vi "Custom Device Express CORE.vi"(8 "error in":errorcluster, 11 "CDEW_MetaDataObj in":refnum<class "NIVS_CDEW_MetaDataObj.lvclass">) -> (0 "error out":errorcluster, 3 "CDEW_MetaDataObj out":refnum<class "NIVS_CDEW_MetaDataObj.lvclass">)   [LabVIEW 2026, in "NIVS_CDEW_MetaDataObj.lvclass"]
doc: "This VI is the Core VI for the Custom Device Wizard.\n\nWritten by:\nStephan Daunke\n\nDate:\n2014/01/27\n\nCompany:\nNational Instruments Germany GmbH"
uses:
  NIVS_CDEW_MetaDataObj.lvclass
  NIVS_CDEW_MetaDataObj.lvclass/NIVS_CDEW_MetaDataObj.ctl
  Support/XML Parser/XML Parser.lvlib
  <vilib>/AppBuilder/AB_API_Simple/NI_App_Builder_API.lvlib
  0d099170-2439-4ee0-9fc1-b5448e48b177.vi
  <vilib>/AppBuilder/AB_API_Simple/Build (path).vi
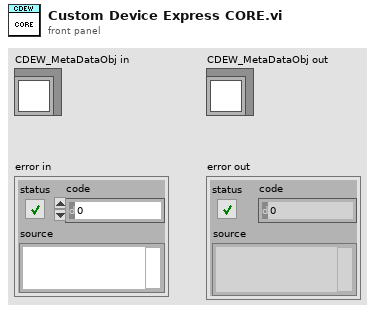
[diagram p1: front panel]
types:
  T1 = enum16{"Create CD Root Folder", "Copy Compiled Settings", "Generate Custom Device DLL from XML", "Calculate Page Properties", "Create Configuration Project", "Create Engine Project", "Create Custom Device Engine Project", "Create System Explorer Project", "Create Test Hooks Project", "Relink and Clean Up VIs", "Build PPLs", "Copy Custom Device DLL to Public Documents", "Open Projects"}
  T2 = enum16{"Create CD Root Folder", "Copy Compiled Settings", "Generate Custom Device DLL from XML", "Calculate Page Properties", "Create Configuration Project", "Create Engine Project", "Create Custom Device Engine Project", "Create System Explorer Project", "Create Test Hooks Project", "Relink and Clean Up VIs", "Build PPLs", "Copy Custom Device DLL to Public Documents", "Open Projects"}[]
  T3 = typedef "NIVS_CDEW_MetaDataObj.lvclass/Page Properties.ctl" = cluster{"Type":T4, "Name":string, "GUID":string, "PageDetail":string, "PageVIPath":path}
  T4 = typedef "NIVS_CDEW_MetaDataObj.lvclass/Page Types.ctl" = enum16{"None", "CustomDevice", "Channel", "Waveform", "Section", "DynamicChannel", "DynamicWaveform", "DynamicSection"}
  T5 = cluster{"Project":path, "Target":string, "BuildSpec":string}[]
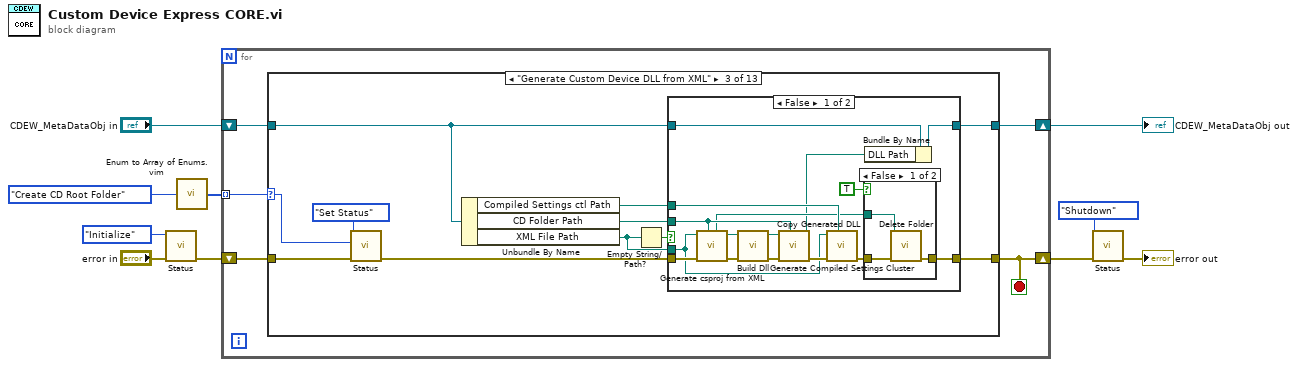
[diagram p0: block diagram]
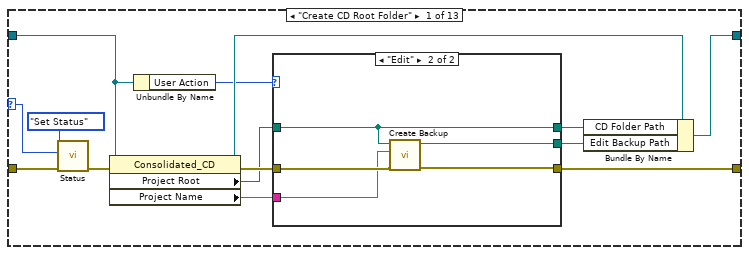
[diagram p2: hidden frame]
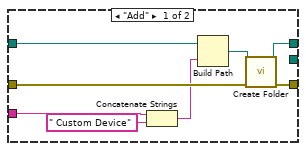
[diagram p3: hidden frame]
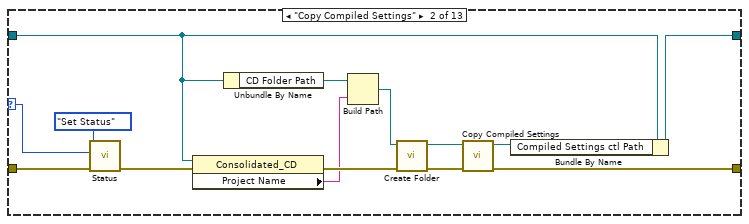
[diagram p4: hidden frame]
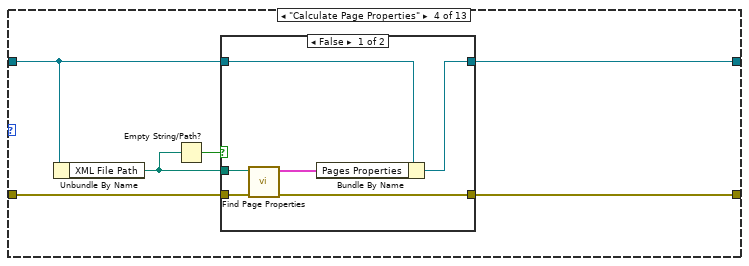
[diagram p7: hidden frame]
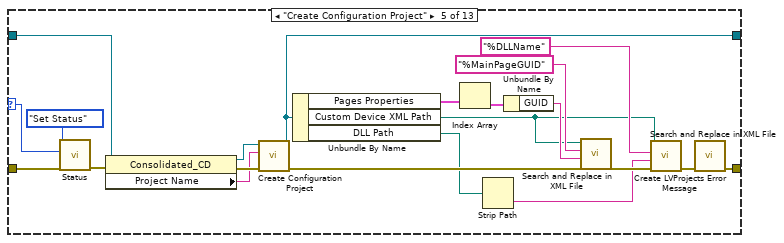
[diagram p9: hidden frame]
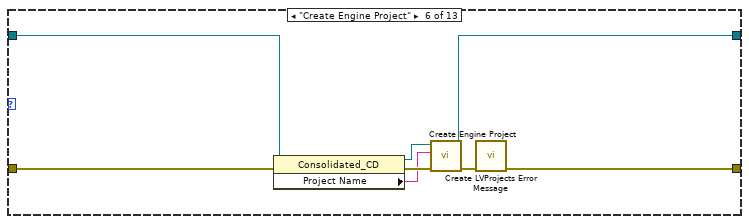
[diagram p10: hidden frame]
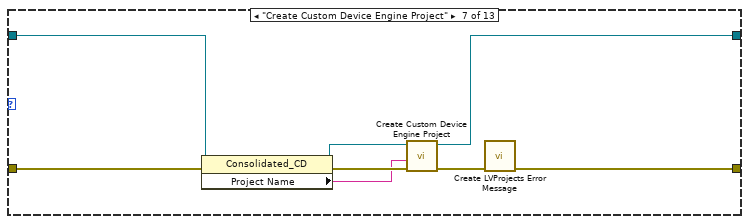
[diagram p11: hidden frame]
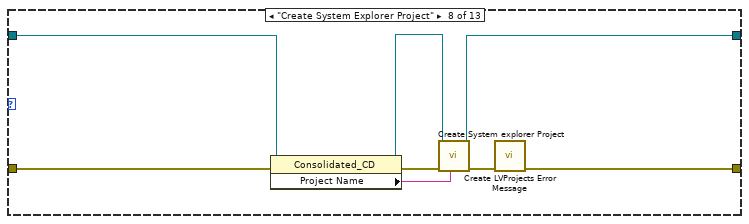
[diagram p12: hidden frame]
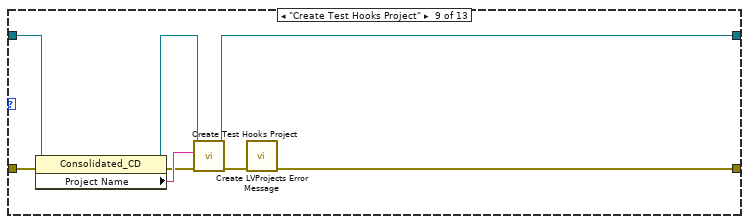
[diagram p13: hidden frame]
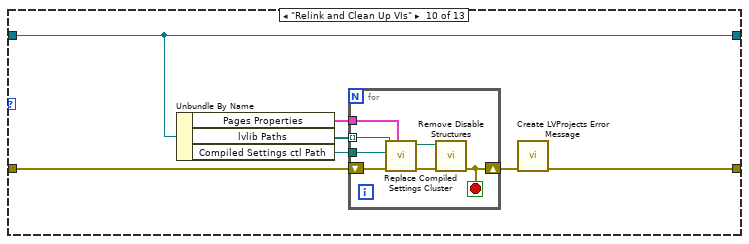
[diagram p14: hidden frame]
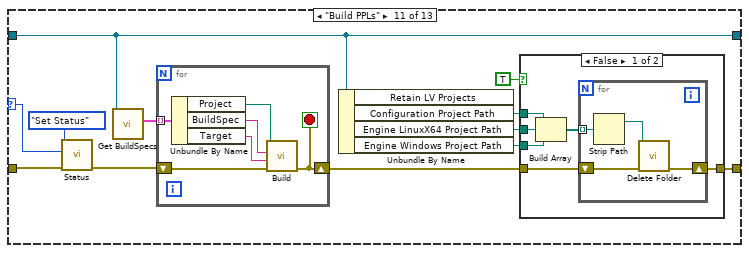
[diagram p15: hidden frame]
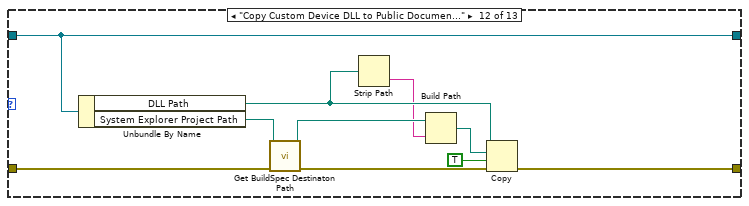
[diagram p17: hidden frame]
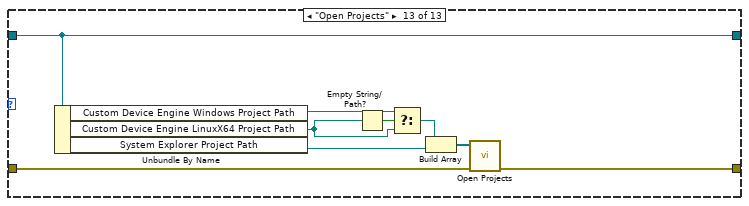
[diagram p18: hidden frame]
diagram:
  n1 = call "Status.vi"("error in"="error in", "Operation"=enum16{"Initialize", "Set Status", "Shutdown"}."Initialize") -> ("error out"=w9:errorcluster)  [unwired: 9 in]
  n2 = call "Enum to Array of Enums.vim"("enum"=T1."Create CD Root Folder") -> ("array of enums"=w1:T2)
  n3 = for {
    shift-right: [w14] -> w8
    shift-left: w9 -> [w15]
    shift-right: [w12] -> w5
    shift-left: "CDEW_MetaDataObj in" -> [w13]
    tunnel: w1 -> [w11] mode=indexing
    stop <- w14 stop-if-true
    n4 = case shown="\"Generate Custom Device DLL from XML\"" w11 {
      selector: w11 -> [w17 w44 w58 _ w105 _ _ _ _ _ w172 _ _]
      tunnel: w15 -> [w27 w53 w66 w95 w119 w131 w139 w147 w156 w163 w180 w207 w218]
      tunnel: [w29 w56 w67 w94 w120 w129 w137 w145 w155 w161 w182 w209 w217] -> w14
      tunnel: w13 -> [w22 w46 w61 w92 w112 w125 w135 w141 w151 w158 w177 w206 w216]
      tunnel: [w23 w51 w60 w93 w116 w127 w134 w143 w154 w158 w177 w206 w216] -> w12
      frame "Create CD Root Folder" {
        n5 = call "Status.vi"("error in"=w27, "State"=w17, "Operation"=enum16{"Initialize", "Set Status", "Shutdown"}."Set Status") -> ("error out"=w26:errorcluster)  [unwired: 8 in]
        n6 = property class="Consolidated_CD"(reference=w22, error in=w26) -> (reference out=w25:refnum<class "NIVS_CDEW_MetaDataObj.lvclass">, error out=w28:errorcluster, "Project Root"=w20:path, "Project Name"=w19:string)
        n7 = Unbundle By Name(w22) -> ("User Action"=w21:enum16{"Add", "Edit"})
        n8 = case shown="\"Edit\"" w21 {
          tunnel: [w37 w41] -> w29
          tunnel: [w35 w38] -> w24
          tunnel: w28 -> [w36 w42]
          tunnel: w20 -> [w33 w38]
          tunnel: w19 -> [w32 w40]
          tunnel: [_ w39] -> w18
          frame "Add" {
            n9 = Concatenate Strings(w32, " Custom Device" ("string")) -> (w30:string)
            n10 = Build Path(base path=w33, name or relative path=w30) -> (appended path=w34:path)
            n11 = call "Create Folder.vi"("error in"=w36, "Folder Path"=w34) -> ("error out"=w37:errorcluster, "Folder Path Out"=w35:path)  [unwired: 8 in]
          }
          frame "Edit" {
            n12 = call "Create Backup.vi"("error in"=w42, "Custom Device Name"=w40, "Custom Device Folder"=w38) -> ("error out"=w41:errorcluster, "Edit Backup Path"=w39:path)  [unwired: 7 in]
          }
        }
        n13 = Bundle By Name(cluster=w25, "CD Folder Path"=w24, "Edit Backup Path"=w18) -> (w23:refnum<class "NIVS_CDEW_MetaDataObj.lvclass">)
      }
      frame "Copy Compiled Settings" {
        n14 = call "Status.vi"("error in"=w53, "State"=w44, "Operation"=enum16{"Initialize", "Set Status", "Shutdown"}."Set Status") -> ("error out"=w52:errorcluster)  [unwired: 8 in]
        n15 = property class="Consolidated_CD"(reference=w46, error in=w52) -> (error out=w54:errorcluster, "Project Name"=w45:string)  [unwired: 1 out]
        n16 = Unbundle By Name(w46) -> ("CD Folder Path"=w49:path)
        n17 = Build Path(base path=w49, name or relative path=w45) -> (appended path=w48:path)
        n18 = call "Create Folder.vi"("error in"=w54, "Folder Path"=w48) -> ("error out"=w55:errorcluster, "Folder Path Out"=w47:path)  [unwired: 8 in]
        n19 = call "Copy Compiled Settings.vi"("error in"=w55, "Custom Device Folder"=w47) -> ("error out"=w56:errorcluster, "Compiled Settings ctl File Path"=w50:path)  [unwired: 8 in]
        n20 = Bundle By Name(cluster=w46, "Compiled Settings ctl Path"=w50) -> (w51:refnum<class "NIVS_CDEW_MetaDataObj.lvclass">)
      }
      frame "Generate Custom Device DLL from XML" {
        n21 = call "Status.vi"("error in"=w66, "State"=w58, "Operation"=enum16{"Initialize", "Set Status", "Shutdown"}."Set Status") -> ("error out"=w65:errorcluster)  [unwired: 8 in]
        n22 = Unbundle By Name(w61) -> ("Compiled Settings ctl Path"=w59:path, "CD Folder Path"=w62:path, "XML File Path"=w64:path)
        n23 = Empty String/Path?(string/path=w64) -> (empty?=w63:bool)
        n24 = case shown="False" w63 {
          tunnel: w65 -> [w83 w89]
          tunnel: [w78 w89] -> w67
          tunnel: w64 -> [w75 _]
          tunnel: w62 -> [w74 _]
          tunnel: w61 -> [w73 w88]
          tunnel: [w70 w88] -> w60
          tunnel: w59 -> [w72 _]
          frame False {
            n25 = call "Generate csproj from XML.vi"("CD Root Folder Path"=w74, "error in"=w83, "XML File Path"=w75) -> ("error out"=w81:errorcluster, "csproj Path"=w77:path, "CD Gen code folder"=w71:path)  [unwired: 6 in]
            n26 = call "Build Dll.vi"("error in"=w81, "csproj Path in"=w77) -> ("error out"=w82:errorcluster, "csproj Path out"=w76:path)  [unwired: 8 in]
            n27 = call "Copy Generated DLL.vi"("CD root folder Path"=w74, "error in"=w82, "csproj Path"=w76) -> ("error out"=w80:errorcluster, "CD DLL Path"=w69:path)  [unwired: 7 in]
            n28 = call "Generate Compiled Settings Cluster.vi"("Compiled Settings Path"=w72, "error in"=w80, "XML Path"=w75) -> ("error out"=w79:errorcluster)  [unwired: 8 in]
            n29 = case shown="False" TRUE {
              tunnel: w79 -> [w85 w87]
              tunnel: w71 -> [w84 _]
              tunnel: [w86 w87] -> w78
              frame False {
                n30 = call "Delete Folder.vi"("error in"=w85, "Folder Path"=w84) -> ("error out"=w86:errorcluster)  [unwired: 8 in, 1 out]
              }
              frame True {
              }
            }
            n31 = Bundle By Name(cluster=w73, "DLL Path"=w69) -> (w70:refnum<class "NIVS_CDEW_MetaDataObj.lvclass">)
          }
          frame True {
          }
        }
      }
      frame "Calculate Page Properties" {
        n32 = Unbundle By Name(w92) -> ("XML File Path"=w91:path)
        n33 = Empty String/Path?(string/path=w91) -> (empty?=w90:bool)
        n34 = case shown="False" w90 {
          tunnel: w95 -> [w101 w103]
          tunnel: [w100 w103] -> w94
          tunnel: w91 -> [w99 _]
          tunnel: [w97 w102] -> w93
          tunnel: w92 -> [w96 w102]
          frame False {
            n35 = call "Find Page Properties.vi"("error in"=w101, "XML File Path"=w99) -> ("error out"=w100:errorcluster, "Pages Properties"=w98:T3[])  [unwired: 8 in]
            n36 = Bundle By Name(cluster=w96, "Pages Properties"=w98) -> (w97:refnum<class "NIVS_CDEW_MetaDataObj.lvclass">)
          }
          frame True {
          }
        }
      }
      frame "Create Configuration Project" {
        n37 = call "Status.vi"("error in"=w119, "State"=w105, "Operation"=enum16{"Initialize", "Set Status", "Shutdown"}."Set Status") -> ("error out"=w118:errorcluster)  [unwired: 8 in]
        n38 = property class="Consolidated_CD"(reference=w112, error in=w118) -> (reference out=w113:refnum<class "NIVS_CDEW_MetaDataObj.lvclass">, error out=w124:errorcluster, "Project Name"=w117:string)
        n39 = call "Create Configuration Project.vi"("error in"=w124, "Custom Device Name"=w117, "CDEW_MetaDataObj in"=w113) -> ("error out"=w123:errorcluster, "CDEW_MetaDataObj out"=w116:refnum<class "NIVS_CDEW_MetaDataObj.lvclass">)  [unwired: 7 in]
        n40 = Unbundle By Name(w116) -> ("Pages Properties"=w115:T3[], "Custom Device XML Path"=w108:path, "DLL Path"=w107:path)
        n41 = Index Array(array=w115) -> (element=w114:T3)  [unwired: 1 in]
        n42 = Strip Path(path=w107) -> (name=w106:string)  [unwired: 1 out]
        n43 = Unbundle By Name(w114) -> ("GUID"=w111:string)
        n44 = call "Search and Replace in XML File.vi"("error in"=w123, "Replace String"=w111, "Search String"="%MainPageGUID" ("search string"), "Custom Device XML Path"=w108) -> ("error out"=w122:errorcluster)  [unwired: 7 in]
        n45 = call "Search and Replace in XML File.vi"("error in"=w122, "Replace String"=w106, "Search String"="%DLLName", "Custom Device XML Path"=w108) -> ("error out"=w121:errorcluster)  [unwired: 7 in]
        n46 = call "Create LVProjects Error Message.vi"("error in"=w121) -> ("error out"=w120:errorcluster)  [unwired: 10 in]
      }
      frame "Create Engine Project" {
        n47 = property class="Consolidated_CD"(reference=w125, error in=w131) -> (reference out=w126:refnum<class "NIVS_CDEW_MetaDataObj.lvclass">, error out=w132:errorcluster, "Project Name"=w128:string)
        n48 = call "Create Engine Project.vi"("error in"=w132, "Custom Device Name"=w128, "CDEW_MetaDataObj in"=w126) -> ("error out"=w130:errorcluster, "CDEW_MetaDataObj out"=w127:refnum<class "NIVS_CDEW_MetaDataObj.lvclass">)  [unwired: 7 in]
        n49 = call "Create LVProjects Error Message.vi"("error in"=w130) -> ("error out"=w129:errorcluster)  [unwired: 10 in]
      }
      frame "Create Custom Device Engine Project" {
        n50 = property class="Consolidated_CD"(reference=w135, error in=w139) -> (reference out=w133:refnum<class "NIVS_CDEW_MetaDataObj.lvclass">, error out=w140:errorcluster, "Project Name"=w136:string)
        n51 = call "Create Custom Device Engine Project.vi"("error in"=w140, "Custom Device Name"=w136, "CDEW_MetaDataObj in"=w133) -> ("error out"=w138:errorcluster, "CDEW_MetaDataObj out"=w134:refnum<class "NIVS_CDEW_MetaDataObj.lvclass">)  [unwired: 7 in]
        n52 = call "Create LVProjects Error Message.vi"("error in"=w138) -> ("error out"=w137:errorcluster)  [unwired: 10 in]
      }
      frame "Create System Explorer Project" {
        n53 = property class="Consolidated_CD"(reference=w141, error in=w147) -> (reference out=w142:refnum<class "NIVS_CDEW_MetaDataObj.lvclass">, error out=w148:errorcluster, "Project Name"=w144:string)
        n54 = call "Create System explorer Project.vi"("Custom Device Name"=w144, "error in"=w148, "CDEW_MetaDataObj in"=w142) -> ("error out"=w146:errorcluster, "CDEW_MetaDataObj out"=w143:refnum<class "NIVS_CDEW_MetaDataObj.lvclass">)  [unwired: 7 in]
        n55 = call "Create LVProjects Error Message.vi"("error in"=w146) -> ("error out"=w145:errorcluster)  [unwired: 10 in]
      }
      frame "Create Test Hooks Project" {
        n56 = property class="Consolidated_CD"(reference=w151, error in=w156) -> (reference out=w152:refnum<class "NIVS_CDEW_MetaDataObj.lvclass">, error out=w150:errorcluster, "Project Name"=w153:string)
        n57 = call "Create Test Hooks Project.vi"("error in"=w150, "CD Name"=w153, "CDEW_MetaDataObj in"=w152) -> ("error out"=w149:errorcluster, "CDEW_MetaDataObj out"=w154:refnum<class "NIVS_CDEW_MetaDataObj.lvclass">)  [unwired: 7 in]
        n58 = call "Create LVProjects Error Message.vi"("error in"=w149) -> ("error out"=w155:errorcluster)  [unwired: 10 in]
      }
      frame "Relink and Clean Up VIs" {
        n59 = Unbundle By Name(w158) -> ("Pages Properties"=w157:T3[], "lvlib Paths"=w160:path[], "Compiled Settings ctl Path"=w159:path)
        n60 = for {
          tunnel: w159 -> [w167]
          tunnel: w160 -> [w166] mode=indexing
          shift-right: [w168] -> w162
          shift-left: w163 -> [w169]
          tunnel: w157 -> [w164]
          stop <- w168 stop-if-true
          n61 = call "Replace Compiled Settings Cluster.vi"("Pages Properties"=w164, "error in"=w169, "Compiled Settings ctl path"=w167, "lvlib path"=w166) -> ("error out"=w170:errorcluster, "lvlib path out"=w165:path)  [unwired: 6 in]
          n62 = call "Remove Disable Structures.vi"("error in"=w170, "lvlib path"=w165) -> ("error out"=w168:errorcluster)  [unwired: 9 in]
        }
        n63 = call "Create LVProjects Error Message.vi"("error in"=w162) -> ("error out"=w161:errorcluster)  [unwired: 10 in]
      }
      frame "Build PPLs" {
        n64 = call "Status.vi"("error in"=w180, "State"=w172, "Operation"=enum16{"Initialize", "Set Status", "Shutdown"}."Set Status") -> ("error out"=w179:errorcluster)  [unwired: 8 in]
        n65 = call "Get BuildSpecs.vi"("CDEW_MetaDataObj"=w177) -> ("Project BuildSpecs with Targets"=w176:T5)  [unwired: 10 in]
        n66 = for {
          tunnel: w176 -> [w186] mode=indexing
          shift-right: [w187] -> w181
          shift-left: w179 -> [w188]
          stop <- w187 stop-if-true
          n67 = Unbundle By Name(w186) -> ("Project"=w185:path, "BuildSpec"=w184:string, "Target"=w183:string)
          n68 = call-poly <vilib>:"Build.vi"("error in (no error)"=w188, "Name of target (My Computer)"=w183, "Name of build specification (if empty: build all)"=w184, "Path to project"=w185) -> ("error out"=w187:errorcluster)  [unwired: 6 in, 1 out]
        }
        n69 = Unbundle By Name(w177) -> ("Configuration Project Path"=w178:path, "Engine LinuxX64 Project Path"=w175:path, "Engine Windows Project Path"=w174:path)  [unwired: 1 out]
        n70 = case shown="False" TRUE {
          tunnel: w181 -> [w194 w199]
          tunnel: [w193 w199] -> w182
          tunnel: w178 -> [w192 _]
          tunnel: w175 -> [w191 _]
          tunnel: w174 -> [w189 _]
          frame False {
            n71 = Build Array(w192, w191, w189) -> (w190:path[])
            n72 = for {
              shift-right: [w197] -> w193
              shift-left: w194 -> [w198]
              tunnel: w190 -> [w196] mode=indexing
              n73 = Strip Path(path=w196) -> (stripped path=w195:path)  [unwired: 1 out]
              n74 = call "Delete Folder.vi"("error in"=w198, "Folder Path"=w195) -> ("error out"=w197:errorcluster)  [unwired: 8 in, 1 out]
            }
          }
          frame True {
          }
        }
      }
      frame "Copy Custom Device DLL to Public Documents" {
        n75 = Unbundle By Name(w206) -> ("DLL Path"=w201:path, "System Explorer Project Path"=w205:path)
        n76 = call "Get BuildSpec Destinaton Path.vi"("error in"=w207, "Project Path"=w205) -> ("error out"=w208:errorcluster, "Build path"=w204:path)  [unwired: 8 in]
        n77 = Strip Path(path=w201) -> (name=w200:string)  [unwired: 1 out]
        n78 = Build Path(base path=w204, name or relative path=w200) -> (appended path=w203:path)
        n79 = Copy(8:w208, 9:TRUE ("overwrite (F)"), 10:w203, 11:w201) -> (0:w209:errorcluster)  [unwired: 1 in, 2 out]
      }
      frame "Open Projects" {
        n80 = Unbundle By Name(w216) -> ("Custom Device Engine Windows Project Path"=w211:path, "Custom Device Engine LinuxX64 Project Path"=w212:path, "System Explorer Project Path"=w214:path)
        n81 = Empty String/Path?(string/path=w212) -> (empty?=w213:bool)
        n82 = Select(t=w211, s=w213, f=w212) -> (s? t:f=w210:path)
        n83 = Build Array(w210, w214) -> (w215:path[])
        n84 = call "Open Projects.vi"("error in"=w218, "Project paths"=w215) -> ("error out"=w217:errorcluster)  [unwired: 9 in]
      }
    }
  }
  "CDEW_MetaDataObj out" <- w5
  n85 = call "Status.vi"("error in"=w8, "Operation"=enum16{"Initialize", "Set Status", "Shutdown"}."Shutdown") -> ("error out"=→"error out":errorcluster)  [unwired: 9 in]
